vi "Update Packages (Diff).vi"(8 "error in (no error)":errorcluster, 11 "Artifactory.VIPM in":refnum<class "Artifactory.VIPM.lvclass">) -> (0 "error out":errorcluster, 2 "Sync'ed Files":path[](array[path]), 3 "Artifactory.VIPM out":refnum<class "Artifactory.VIPM.lvclass">)   [LabVIEW 2021, in "Artifactory.VIPM.lvclass"]
uses:
  Artifactory.VIPM.lvclass
  C:/Repositories/LVOS/Artifactory/lv-src/Artifactory/Artifactory.lvclass
  Artifactory/Artifactory.lvclass/Artifactory.ctl
  Artifactory.VIPM.lvclass/Artifactory.VIPM.ctl
  Artifactory/Artifactory.lvclass
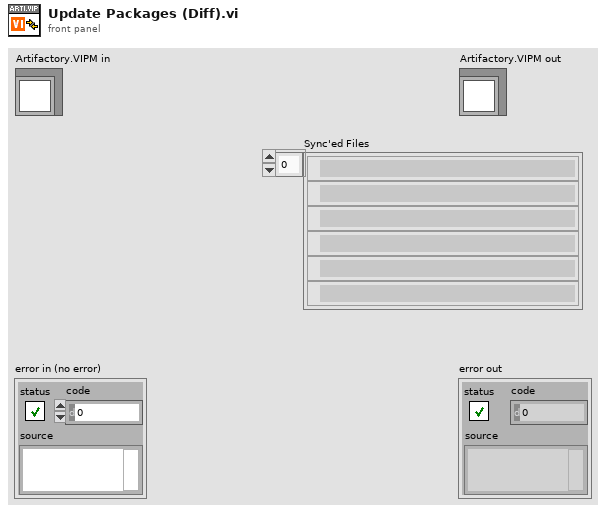
[diagram p1: front panel]
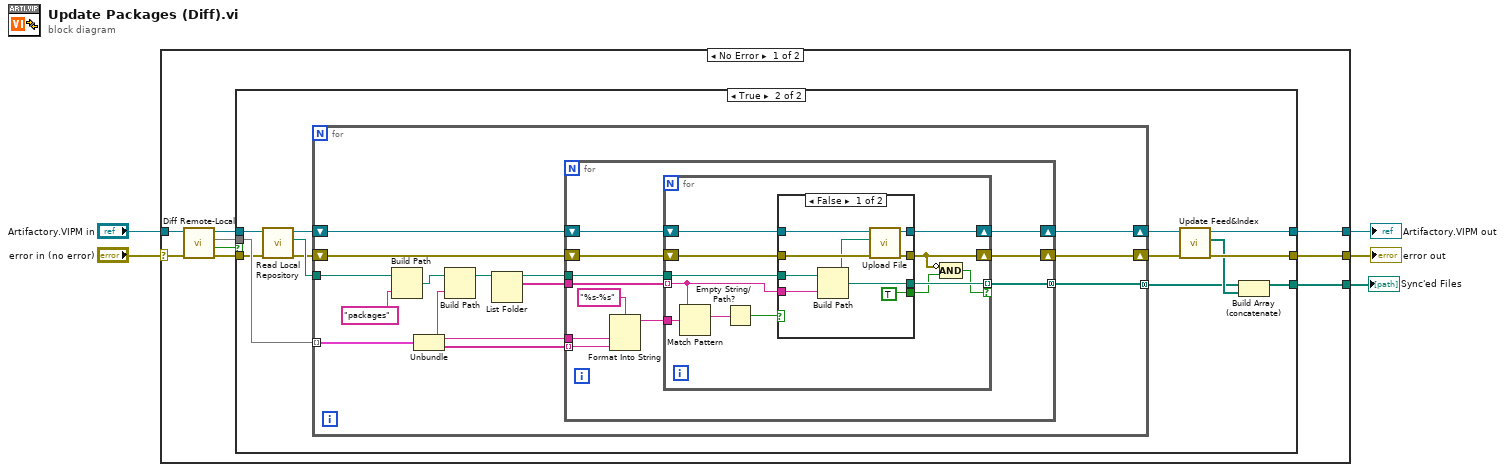
[diagram p0: block diagram]
diagram:
  n1 = case shown="No Error" "error in (no error)" {
    selector: "error in (no error)" -> [w11 w77]
    tunnel: [w13 w77] -> w4
    tunnel: [w14 w76] -> w2
    tunnel: "Artifactory.VIPM in" -> [w12 w76]
    tunnel: [w6 _] -> w1
    frame No Error {
      n2 = call "Diff Remote-Local.vi"("error in (no error)"=w11, "Artifactory.VIPM in"=w12) -> ("error out"=w10:errorcluster, "has Changes?"=w8:bool, "DIff"=w7:map{string, string[]}, "Artifactory.VIPM out"=w9:refnum<class "Artifactory.VIPM.lvclass">)  [unwired: 6 in]
      n3 = case shown="True" w8 {
        tunnel: [w16 w23] -> w14
        tunnel: [w15 w24] -> w13
        tunnel: w10 -> [w15 w17]
        tunnel: w9 -> [w16 w27]
        tunnel: w7 -> [_ w22]
        tunnel: [_ w18] -> w6
        frame False {
        }
        frame True {
          n4 = call "Read Local Repository.vi"("Artifactory in"=w27) -> ("Local Repository"=w21:path, "Artifactory out"=w28:refnum<class "Artifactory.VIPM.lvclass">)  [unwired: 9 in]
          n5 = for {
            shift-right: [w41] -> w26
            shift-left: w28 -> [w42]
            shift-right: [w39] -> w25
            shift-left: w17 -> [w40]
            tunnel: w21 -> [w30]
            tunnel: w22 -> [w38] mode=indexing
            tunnel: [w36] -> w19 mode=concatenating
            n6 = Build Path(base path=w30, name or relative path="packages" ("format string")) -> (appended path=w31:path)
            n7 = Unbundle(w38) -> ("package_name"=w32:string, "versions"=w37:string[])
            n8 = Build Path(base path=w31, name or relative path=w32) -> (appended path=w35:path)
            n9 = List Folder(path=w35) -> (path out=w34:path, filenames=w33:string[])  [unwired: 3 in, 2 out]
            n10 = for {
              tunnel: w34 -> [w48]
              shift-right: [w52] -> w41
              shift-left: w42 -> [w53]
              shift-right: [w50] -> w39
              shift-left: w40 -> [w51]
              tunnel: w37 -> [w46] mode=indexing
              tunnel: [w49] -> w36 mode=concatenating
              tunnel: w33 -> [w44]
              tunnel: w32 -> [w47]
              n11 = Format Into String(format string="%s-%s", w47, w46) -> (resulting string=w43:string)  [unwired: 2 in, 1 out]
              n12 = for {
                shift-right: [w64] -> w52
                shift-left: w53 -> [w65]
                shift-right: [w56] -> w50
                shift-left: w51 -> [w63]
                tunnel: w48 -> [w62]
                tunnel: [w61] -> w49 mode=indexing if=w54
                tunnel: w44 -> [w59] mode=indexing
                tunnel: w43 -> [w60]
                n13 = Match Pattern(string=w59, regular expression=w60) -> (match substring=w58:string)  [unwired: 1 in, 3 out]
                n14 = Empty String/Path?(string/path=w58) -> (empty?=w57:bool)
                n15 = case shown="False" w57 {
                  tunnel: w65 -> [w73 w75]
                  tunnel: [w72 w75] -> w64
                  tunnel: w63 -> [w71 w74]
                  tunnel: [w70 w74] -> w56
                  tunnel: w62 -> [w69 _]
                  tunnel: [w68 _] -> w61
                  tunnel: w59 -> [w67 _]
                  tunnel: [TRUE _] -> w55
                  frame False {
                    n16 = Build Path(base path=w69, name or relative path=w67) -> (appended path=w68:path)
                    n17 = call "Upload File.vi"("error in (no error)"=w71, "Local File"=w68, "Artifactory in"=w73) -> ("error out"=w70:errorcluster, "Artifactory out"=w72:refnum<class "Artifactory.VIPM.lvclass">)  [unwired: 7 in]
                  }
                  frame True {
                  }
                }
                n18 = Compound Arithmetic op=AND(invert w56, w55) -> (w54:bool)
              }
            }
          }
          n19 = call "Update Feed&Index.vi"("error in (no error)"=w25, "Artifactory.VIPM in"=w26) -> ("error out"=w24:errorcluster, "Sync'ed Files"=w20:path[], "Artifactory.VIPM out"=w23:refnum<class "Artifactory.VIPM.lvclass">)  [unwired: 7 in]
          n20 = Build Array (concatenate)(w19, w20) -> (w18:path[])
        }
      }
    }
    frame Error {
    }
  }
  "error out" <- w4
  "Artifactory.VIPM out" <- w2
  "Sync'ed Files" <- w1
